vi "Main.vi"() -> ()   [LabVIEW 2018] (continued)
                n297 = case shown="真" w8265 {
                  tunnel: w8264 -> [_ w8271]
                  tunnel: w8263 -> [w8267 w8270]
                  tunnel: [w8267 w8269] -> _
                  frame False {
                  }
                  frame True {
                    n298 = flat-sequence {
                      tunnel: [w8274] -> w8272
                      tunnel: w8271 -> [w8273]
                      tunnel: w8270 -> [w8275]
                      tunnel: [w8273] -> w8268
                      tunnel: w8272 -> [w8305]
                      tunnel: [w8297] -> w8269
                      tunnel: w8268 -> [w8289]
                      frame #0 {
                        n299 = call "EXCEL 画曲线.vi"("错误输入（无错误）"=w8275, "路径"=w8273) -> ("error IO"=w8274:errorcluster, "XY图"=→"ST70_R曲线":cluster{"X":dbl, "Y":dbl}[])  [unwired: 6 in, 2 out]
                      }
                      frame #1 {
                        w8285 = path "D:/Data_Storage/temp" ("appended path")
                        n300 = local read "70编码"() -> (w8284:string)
                        n301 = call <vilib>:"Check if File or Folder Exists.vi"("path"=w8285) -> ("error out"=w8299:errorcluster, "file or folder exists?"=w8298:bool)  [unwired: 8 in, 1 out]
                        n302 = case shown="假" w8298 {
                          tunnel: w8285 -> [w8322 w8324]
                          tunnel: [w8321 w8324] -> w8291
                          tunnel: w8299 -> [w8320 w8323]
                          tunnel: [w8319 w8323] -> w8292
                          frame False {
                            n303 = Create Folder(path (use dialog)=w8322, error in=w8320) -> (created path=w8321:path, error out=w8319:errorcluster)  [unwired: 1 in, 1 out]
                          }
                          frame True {
                          }
                        }
                        n304 = Concatenate Strings(w8284, "ST70_R.BMP" ("字符串")) -> (w8302:string)
                        n305 = Build Path(base path=w8291, name or relative path=w8284) -> (appended path=w8293:path)
                        n306 = call <vilib>:"Check if File or Folder Exists.vi"("error in (no error)"=w8292, "path"=w8293) -> ("error out"=w8294:errorcluster, "file or folder exists?"=w8295:bool)  [unwired: 7 in, 1 out]
                        n307 = case shown="假" w8295 {
                          tunnel: w8293 -> [w8316 w8318]
                          tunnel: [w8315 w8318] -> w8280
                          tunnel: w8294 -> [w8314 w8317]
                          tunnel: [w8313 w8317] -> w8278
                          frame False {
                            n308 = Create Folder(path (use dialog)=w8316, error in=w8314) -> (created path=w8315:path, error out=w8313:errorcluster)  [unwired: 1 in, 1 out]
                          }
                          frame True {
                          }
                        }
                        n309 = Build Path(base path=w8280, name or relative path="ST70R" ("名称或相对路径")) -> (appended path=w8283:path)
                        n310 = call <vilib>:"Check if File or Folder Exists.vi"("error in (no error)"=w8278, "path"=w8283) -> ("error out"=w8282:errorcluster, "file or folder exists?"=w8281:bool)  [unwired: 7 in, 1 out]
                        n311 = case shown="假" w8281 {
                          tunnel: w8283 -> [w8310 w8312]
                          tunnel: [w8309 w8312] -> w8277
                          tunnel: w8282 -> [w8308 w8311]
                          tunnel: [w8307 w8311] -> _
                          frame False {
                            n312 = Create Folder(path (use dialog)=w8310, error in=w8308) -> (created path=w8309:path, error out=w8307:errorcluster)  [unwired: 1 in, 1 out]
                          }
                          frame True {
                          }
                        }
                        n313 = Build Path(base path=w8277, name or relative path=w8302) -> (appended path=w8288:path)
                        n314 = call "文件路径.vi"("文件路径"=w8288, "文件格式"=".BMP") -> ("新路径"=w8287:path)  [unwired: 9 in]
                        n315 = invoke on="ST70_R曲线" class="XYGraph (严格)" method="Export Image"(error in=w8305, "FileType"=enum32{"BMP", "EPS", "EMF", "PICT"}."BMP" ("文件类型"), "Target"=enum32{"File", "Clipboard"}."File" ("目标"), "Path"=w8287, "HideGrid"=FALSE ("隐藏网格"), "Overwrite"=TRUE ("隐藏网格")) -> (error out=w8290:errorcluster)  [unwired: 2 in, 7 out]
                        n316 = Move(source path=w8289, error in=w8290, 9:TRUE ("覆盖(F)"), 10:w8277) -> (error out=w8297:errorcluster)  [unwired: 1 in, 2 out]
                      }
                    }
                  }
                }
              }
              frame #1 {
                n317 = call "检查曲线文件.vi"("Folder Path"=path "D:/op70" ("路径")) -> ("Error Out"=w8327:errorcluster, "Exit?"=w8329:bool, "曲线文件路径"=w8328:path)  [unwired: 7 in, 1 out]
                n318 = case shown="真" w8329 {
                  tunnel: w8328 -> [_ w8334]
                  tunnel: w8327 -> [w8330 w8333]
                  tunnel: [w8330 w8332] -> w8325
                  frame False {
                  }
                  frame True {
                    n319 = flat-sequence {
                      tunnel: [w8337] -> w8335
                      tunnel: w8334 -> [w8336]
                      tunnel: w8333 -> [w8338]
                      tunnel: [w8336] -> w8331
                      tunnel: w8335 -> [w8369]
                      tunnel: [w8364] -> w8332
                      tunnel: w8331 -> [w8361]
                      frame #0 {
                        n320 = call "EXCEL 画曲线.vi"("错误输入（无错误）"=w8338, "路径"=w8336) -> ("error IO"=w8337:errorcluster, "XY图"=→"ST70_L曲线":cluster{"X":dbl, "Y":dbl}[])  [unwired: 6 in, 2 out]
                      }
                      frame #1 {
                        w8352 = path "D:/Data_Storage/temp" ("appended path")
                        n321 = local read "70编码"() -> (w8351:string)
                        n322 = call <vilib>:"Check if File or Folder Exists.vi"("path"=w8352) -> ("error out"=w8359:errorcluster, "file or folder exists?"=w8358:bool)  [unwired: 8 in, 1 out]
                        n323 = case shown="假" w8358 {
                          tunnel: w8352 -> [w8385 w8387]
                          tunnel: [w8384 w8387] -> w8353
                          tunnel: w8359 -> [w8383 w8386]
                          tunnel: [w8382 w8386] -> w8354
                          frame False {
                            n324 = Create Folder(path (use dialog)=w8385, error in=w8383) -> (created path=w8384:path, error out=w8382:errorcluster)  [unwired: 1 in, 1 out]
                          }
                          frame True {
                          }
                        }
                        n325 = Concatenate Strings(w8351, "ST70_L.BMP" ("字符串")) -> (w8340:string)
                        n326 = Build Path(base path=w8353, name or relative path=w8351) -> (appended path=w8355:path)
                        n327 = call <vilib>:"Check if File or Folder Exists.vi"("error in (no error)"=w8354, "path"=w8355) -> ("error out"=w8356:errorcluster, "file or folder exists?"=w8357:bool)  [unwired: 7 in, 1 out]
                        n328 = case shown="假" w8357 {
                          tunnel: w8355 -> [w8379 w8381]
                          tunnel: [w8378 w8381] -> w8347
                          tunnel: w8356 -> [w8377 w8380]
                          tunnel: [w8376 w8380] -> w8345
                          frame False {
                            n329 = Create Folder(path (use dialog)=w8379, error in=w8377) -> (created path=w8378:path, error out=w8376:errorcluster)  [unwired: 1 in, 1 out]
                          }
                          frame True {
                          }
                        }
                        n330 = Build Path(base path=w8347, name or relative path="ST70L" ("名称或相对路径")) -> (appended path=w8350:path)
                        n331 = call <vilib>:"Check if File or Folder Exists.vi"("error in (no error)"=w8345, "path"=w8350) -> ("error out"=w8349:errorcluster, "file or folder exists?"=w8348:bool)  [unwired: 7 in, 1 out]
                        n332 = case shown="假" w8348 {
                          tunnel: w8350 -> [w8373 w8375]
                          tunnel: [w8372 w8375] -> w8342
                          tunnel: w8349 -> [w8371 w8374]
                          tunnel: [w8370 w8374] -> _
                          frame False {
                            n333 = Create Folder(path (use dialog)=w8373, error in=w8371) -> (created path=w8372:path, error out=w8370:errorcluster)  [unwired: 1 in, 1 out]
                          }
                          frame True {
                          }
                        }
                        n334 = Build Path(base path=w8342, name or relative path=w8340) -> (appended path=w8344:path)
                        n335 = call "文件路径.vi"("文件路径"=w8344, "文件格式"=".BMP") -> ("新路径"=w8341:path)  [unwired: 9 in]
                        n336 = invoke on="ST70_L曲线" class="XYGraph (严格)" method="Export Image"(error in=w8369, "FileType"=enum32{"BMP", "EPS", "EMF", "PICT"}."BMP" ("文件类型"), "Target"=enum32{"File", "Clipboard"}."File" ("目标"), "Path"=w8341, "HideGrid"=FALSE ("隐藏网格"), "Overwrite"=TRUE ("隐藏网格")) -> (error out=w8362:errorcluster)  [unwired: 2 in, 7 out]
                        n337 = Move(source path=w8361, error in=w8362, 9:TRUE ("覆盖(F)"), 10:w8342) -> (error out=w8364:errorcluster)  [unwired: 1 in, 2 out]
                      }
                    }
                  }
                }
              }
            }
            n338 = case shown="错误" w8261 {
              selector: w8261 -> [_ w8396]
              frame No Error {
                w8390 = path "D:/op70" ("路径")
                n339 = List Folder(path=w8390) -> (filenames=w8391:string[])  [unwired: 3 in, 3 out]
                n340 = local write "数据保存请求回复70"("1" ("数据保存请求回复70")) -> ()
                n341 = local write "70数据回复输入"(TRUE) -> ()
                n342 = for {
                  tunnel: w8391 -> [w8394] mode=indexing
                  tunnel: w8390 -> [w8395]
                  n343 = Build Path(base path=w8395, name or relative path=w8394) -> (appended path=w8392:path)
                  n344 = Delete(path (use dialog)=w8392, entire hierarchy (F)=TRUE ("整个层次结构(F)")) -> ()  [unwired: 3 in, 3 out]
                }
              }
              frame Error {
                n345 = stacked-sequence {
                  tunnel: w8396 -> [w8402]
                  frame #0 {
                    n346 = Unbundle By Name(w8402) -> ("source"=w8401:string)
                    n347 = local write "数据保存请求回复70"("1" ("数据保存请求回复70")) -> ()
                    n348 = property on="错误信息" class="LstBox (严格)"() -> ("Item Names"=w8408:string[])  [unwired: 2 in, 2 out]
                    n349 = Format Date/Time String(time format string (%c)="%Y-%m-%d %H:%M:%S" ("时间格式字符串(%c)")) -> (date/time string=w8403:string)  [unwired: 2 in]
                    n350 = Concatenate Strings(w8403, "---" ("字符串"), w8401) -> (w8399:string)
                    n351 = Concatenate Strings(w8399, "  " ("字符串"), "ST70 画曲线错误") -> (w8406:string)
                    n352 = local write "70数据回复输入"(TRUE) -> ()
                    n353 = Insert Into Array(array=w8408, index=0 ("索引"), new element=w8406) -> (w8405:string[])
                    n354 = property on="错误信息" class="LstBox (严格)"("Item Names"=w8405) -> ()  [unwired: 2 in, 2 out]
                  }
                }
              }
            }
            "ST70画曲线" <- FALSE ("ST70画曲线")
          }
          event "ST90画曲线": Value Change {
            n355 = event-data() -> ()  [unwired: 1 in, 3 out]
            n356 = stacked-sequence {
              seq-local: [w8413 _ _ _ _ _] -> [_ _ _ _ _ w8717]
              seq-local: [_ w8481 _ _ _ _] -> [_ _ _ _ _ w8716]
              seq-local: [_ _ w8539 _ _ _] -> [_ _ _ _ _ w8715]
              seq-local: [_ _ _ w8597 _ _] -> [_ _ _ _ _ w8714]
              seq-local: [_ _ _ _ w8655 _] -> [_ _ _ _ _ w8713]
              frame #0 {
                w8415 = "ST70R" ("名称或相对路径")
                w8417 = path "D:/Data_Storage/temp" ("appended path")
                w8420 = path "D:/Data_Storage/temp" ("appended path")
                n357 = local read "901二维码"() -> (w8434:string)
                n358 = call "图片保存.vi"("一维码"=w8434) -> ("dup path"=w8435:path)  [unwired: 9 in, 1 out]
                n359 = Build Path(base path=w8435, name or relative path=w8434) -> (appended path=w8431:path)
                n360 = call <vilib>:"Check if File or Folder Exists.vi"("path"=w8431) -> ("error out"=w8433:errorcluster, "file or folder exists?"=w8432:bool)  [unwired: 8 in, 1 out]
                n361 = case shown="假" w8432 {
                  tunnel: w8431 -> [w8478 w8480]
                  tunnel: [w8477 w8480] -> w8421
                  tunnel: w8433 -> [w8476 w8479]
                  tunnel: [w8475 w8479] -> w8426
                  frame False {
                    n362 = Create Folder(path (use dialog)=w8478, error in=w8476) -> (created path=w8477:path, error out=w8475:errorcluster)  [unwired: 1 in, 1 out]
                  }
                  frame True {
                  }
                }
                n363 = local read "901编码"() -> (w8419:string)
                n364 = Build Path(base path=w8420, name or relative path=w8419) -> (appended path=w8430:path)
                n365 = Build Path(base path=w8430, name or relative path="ST70L" ("名称或相对路径")) -> (appended path=w8427:path)
                n366 = Move(source path=w8427, error in=w8426, 9:TRUE ("覆盖(F)"), 10:w8421) -> (error out=w8422:errorcluster)  [unwired: 1 in, 2 out]
                n367 = case shown="错误" w8422 {
                  tunnel: [errorcluster {"status"=FALSE, "code"=0, "source"=""} ("error out") w8460] -> w8412
                  tunnel: w8421 -> [w8455 w8457]
                  tunnel: w8420 -> [_ w8459]
                  tunnel: w8419 -> [_ w8458]
                  tunnel: [w8455 w8457] -> w8414
                  frame No Error {
                  }
                  frame Error {
                    n368 = Build Path(base path=w8459, name or relative path=w8458) -> (appended path=w8464:path)
                    n369 = Build Path(base path=w8464, name or relative path="ST70L" ("名称或相对路径")) -> (appended path=w8461:path)
                    n370 = Move(source path=w8461, 9:TRUE ("覆盖(F)"), 10:w8457) -> (error out=w8460:errorcluster)  [unwired: 2 in, 2 out]
                  }
                }
                n371 = local read "901编码"() -> (w8416:string)
                n372 = Build Path(base path=w8417, name or relative path=w8416) -> (appended path=w8425:path)
                n373 = Build Path(base path=w8425, name or relative path=w8415) -> (appended path=w8423:path)
                n374 = Move(source path=w8423, 9:TRUE ("覆盖(F)"), 10:w8414) -> (error out=w8418:errorcluster)  [unwired: 2 in, 2 out]
                n375 = case shown="错误" w8418 {
                  tunnel: w8417 -> [_ w8453]
                  tunnel: w8416 -> [_ w8452]
                  tunnel: w8415 -> [_ w8451]
                  tunnel: w8414 -> [_ w8448]
                  tunnel: [errorcluster {"status"=FALSE, "code"=0, "source"=""} ("error out") w8447] -> w8413
                  frame No Error {
                  }
                  frame Error {
                    n376 = Build Path(base path=w8453, name or relative path=w8452) -> (appended path=w8454:path)
                    n377 = Build Path(base path=w8454, name or relative path=w8451) -> (appended path=w8450:path)
                    n378 = Move(source path=w8450, 9:TRUE ("覆盖(F)"), 10:w8448) -> (error out=w8447:errorcluster)  [unwired: 2 in, 2 out]
                  }
                }
                n379 = case shown="错误" w8413 {
                  selector: w8413 -> [_ w8466]
                  frame No Error {
                  }
                  frame Error {
                    w8467 = "  " ("字符串")
                    n380 = Unbundle By Name(w8466) -> ("source"=w8465:string)
                    n381 = property on="错误信息" class="LstBox (严格)"() -> ("Item Names"=w8472:string[])  [unwired: 2 in, 2 out]
                    n382 = Format Date/Time String(time format string (%c)="%Y-%m-%d %H:%M:%S" ("时间格式字符串(%c)")) -> (date/time string=w8473:string)  [unwired: 2 in]
                    n383 = Concatenate Strings(w8473, w8467, "ST90 转移曲线失败ST70R", w8467, w8465) -> (w8470:string)
                    n384 = Insert Into Array(array=w8472, index=0 ("索引"), new element=w8470) -> (w8469:string[])
                    n385 = property on="错误信息" class="LstBox (严格)"("Item Names"=w8469) -> ()  [unwired: 2 in, 2 out]
                  }
                }
                n386 = case shown="错误" w8412 {
                  selector: w8412 -> [_ w8439]
                  frame No Error {
                  }
                  frame Error {
                    w8440 = "  " ("字符串")
                    n387 = Unbundle By Name(w8439) -> ("source"=w8438:string)
                    n388 = property on="错误信息" class="LstBox (严格)"() -> ("Item Names"=w8437:string[])  [unwired: 2 in, 2 out]
                    n389 = Format Date/Time String(time format string (%c)="%Y-%m-%d %H:%M:%S" ("时间格式字符串(%c)")) -> (date/time string=w8444:string)  [unwired: 2 in]
                    n390 = Concatenate Strings(w8444, w8440, "ST90 转移曲线失败ST70L", w8440, w8438) -> (w8442:string)
                    n391 = Insert Into Array(array=w8437, index=0 ("索引"), new element=w8442) -> (w8436:string[])
                    n392 = property on="错误信息" class="LstBox (严格)"("Item Names"=w8436) -> ()  [unwired: 2 in, 2 out]
                  }
                }
              }
              frame #1 {
                n393 = flat-sequence {
                  tunnel: [w8485] -> w8483
                  tunnel: [w8484] -> w8482
                  tunnel: w8483 -> [w8493]
                  tunnel: w8482 -> [w8502]
                  tunnel: [w8491] -> w8481
                  frame #0 {
                    n394 = local read "901二维码"() -> (w8484:string)
                    n395 = Concatenate Strings("D:\\BOSCH\\OP90\\CH_00_1\\PRG_00\\Ch_", w8484, "_001", "______.txt" ("字符串")) -> (w8488:string)
                    n396 = String To Path(string=w8488) -> (path=w8485:path)
                    n397 = call "140画曲线.vi"("文件（使用对话框）"=w8485) -> ("压机旋铆位移压力图"=→"压机旋铆位移压力图_1":cluster{dbl[], dbl[]})  [unwired: 10 in]
                  }
                  frame #1 {
                    n398 = call "图片保存.vi"("一维码"=w8502) -> ("dup path"=w8503:path)  [unwired: 9 in, 1 out]
                    n399 = Build Path(base path=w8503, name or relative path=w8502) -> (appended path=w8518:path)
                    n400 = call <vilib>:"Check if File or Folder Exists.vi"("path"=w8518) -> ("error out"=w8516:errorcluster, "file or folder exists?"=w8517:bool)  [unwired: 8 in, 1 out]
                    n401 = case shown="假" w8517 {
                      tunnel: w8518 -> [w8536 w8538]
                      tunnel: [w8535 w8538] -> w8512
                      tunnel: w8516 -> [w8534 w8537]
                      tunnel: [w8533 w8537] -> w8510
                      frame False {
                        n402 = Create Folder(path (use dialog)=w8536, error in=w8534) -> (created path=w8535:path, error out=w8533:errorcluster)  [unwired: 1 in, 1 out]
                      }
                      frame True {
                      }
                    }
                    n403 = Build Path(base path=w8512, name or relative path="ST901" ("名称或相对路径")) -> (appended path=w8513:path)
                    n404 = call <vilib>:"Check if File or Folder Exists.vi"("error in (no error)"=w8510, "path"=w8513) -> ("error out"=w8514:errorcluster, "file or folder exists?"=w8515:bool)  [unwired: 7 in, 1 out]
                    n405 = case shown="假" w8515 {
                      tunnel: w8513 -> [w8530 w8532]
                      tunnel: [w8529 w8532] -> w8507
                      tunnel: w8514 -> [w8528 w8531]
                      tunnel: [w8527 w8531] -> w8501
                      frame False {
                        n406 = Create Folder(path (use dialog)=w8530, error in=w8528) -> (created path=w8529:path, error out=w8527:errorcluster)  [unwired: 1 in, 1 out]
                      }
                      frame True {
                      }
                    }
                    n407 = Concatenate Strings("Ch_" ("字符串"), w8502, "_001______.txt" ("字符串")) -> (w8504:string)
                    n408 = Concatenate Strings(w8502, "_ST901_001.BMP" ("字符串")) -> (w8508:string)
                    n409 = Build Path(base path=w8507, name or relative path=w8508) -> (appended path=w8498:path)
                    n410 = Build Path(base path=w8507, name or relative path=w8504) -> (appended path=w8492:path)
                    n411 = invoke on="压机旋铆位移压力图_1" class="XYGraph (严格)" method="Export Image"(error in=w8501, "FileType"=enum32{"BMP", "EPS", "EMF", "PICT"}."BMP" ("文件类型"), "Target"=enum32{"File", "Clipboard"}."File" ("目标"), "Path"=w8498, "HideGrid"=FALSE ("隐藏网格"), "Overwrite"=TRUE ("始终覆盖")) -> (error out=w8494:errorcluster)  [unwired: 2 in, 7 out]
                    n412 = Move(source path=w8493, error in=w8494, 9:TRUE ("覆盖(F)"), 10:w8492) -> (error out=w8491:errorcluster)  [unwired: 1 in, 2 out]
                    n413 = case shown="错误" w8491 {
                      frame No Error {
                      }
                      frame Error {
                        n414 = property on="错误信息" class="LstBox (严格)"() -> ("Item Names"=w8523:string[])  [unwired: 2 in, 2 out]
                        n415 = Format Date/Time String(time format string (%c)="%Y-%m-%d %H:%M:%S" ("时间格式字符串(%c)")) -> (date/time string=w8525:string)  [unwired: 2 in]
                        n416 = Concatenate Strings(w8525, "  " ("字符串"), "ST901 画曲线错误") -> (w8521:string)
                        n417 = Insert Into Array(array=w8523, index=0 ("索引"), new element=w8521) -> (w8520:string[])
                        n418 = property on="错误信息" class="LstBox (严格)"("Item Names"=w8520) -> ()  [unwired: 2 in, 2 out]
                      }
                    }
                  }
                }
              }
              frame #2 {
                n419 = flat-sequence {
                  tunnel: [w8543] -> w8541
                  tunnel: [w8542] -> w8540
                  tunnel: w8541 -> [w8551]
                  tunnel: w8540 -> [w8560]
                  tunnel: [w8549] -> w8539
                  frame #0 {
                    n420 = local read "901二维码"() -> (w8542:string)
                    n421 = Concatenate Strings("D:\\BOSCH\\OP90\\CH_00_1\\PRG_00\\Ch_", w8542, "_002", "______.txt" ("字符串")) -> (w8546:string)
                    n422 = String To Path(string=w8546) -> (path=w8543:path)
                    n423 = call "140画曲线.vi"("文件（使用对话框）"=w8543) -> ("压机旋铆位移压力图"=→"压机旋铆位移压力图_2":cluster{dbl[], dbl[]})  [unwired: 10 in]
                  }
                  frame #1 {
                    n424 = call "图片保存.vi"("一维码"=w8560) -> ("dup path"=w8561:path)  [unwired: 9 in, 1 out]
                    n425 = Build Path(base path=w8561, name or relative path=w8560) -> (appended path=w8576:path)
                    n426 = call <vilib>:"Check if File or Folder Exists.vi"("path"=w8576) -> ("error out"=w8574:errorcluster, "file or folder exists?"=w8575:bool)  [unwired: 8 in, 1 out]
                    n427 = case shown="假" w8575 {
                      tunnel: w8576 -> [w8594 w8596]
                      tunnel: [w8593 w8596] -> w8570
                      tunnel: w8574 -> [w8592 w8595]
                      tunnel: [w8591 w8595] -> w8568
                      frame False {
                        n428 = Create Folder(path (use dialog)=w8594, error in=w8592) -> (created path=w8593:path, error out=w8591:errorcluster)  [unwired: 1 in, 1 out]
                      }
                      frame True {
                      }
                    }
                    n429 = Build Path(base path=w8570, name or relative path="ST901" ("名称或相对路径")) -> (appended path=w8571:path)
                    n430 = call <vilib>:"Check if File or Folder Exists.vi"("error in (no error)"=w8568, "path"=w8571) -> ("error out"=w8572:errorcluster, "file or folder exists?"=w8573:bool)  [unwired: 7 in, 1 out]
                    n431 = case shown="假" w8573 {
                      tunnel: w8571 -> [w8588 w8590]
                      tunnel: [w8587 w8590] -> w8565
                      tunnel: w8572 -> [w8586 w8589]
                      tunnel: [w8585 w8589] -> w8559
                      frame False {
                        n432 = Create Folder(path (use dialog)=w8588, error in=w8586) -> (created path=w8587:path, error out=w8585:errorcluster)  [unwired: 1 in, 1 out]
                      }
                      frame True {
                      }
                    }
                    n433 = Concatenate Strings("Ch_" ("字符串"), w8560, "_002______.txt" ("字符串")) -> (w8562:string)
                    n434 = Concatenate Strings(w8560, "_ST901_002.BMP" ("字符串")) -> (w8566:string)
                    n435 = Build Path(base path=w8565, name or relative path=w8566) -> (appended path=w8556:path)
                    n436 = Build Path(base path=w8565, name or relative path=w8562) -> (appended path=w8550:path)
                    n437 = invoke on="压机旋铆位移压力图_2" class="XYGraph (严格)" method="Export Image"(error in=w8559, "FileType"=enum32{"BMP", "EPS", "EMF", "PICT"}."BMP" ("文件类型"), "Target"=enum32{"File", "Clipboard"}."File" ("目标"), "Path"=w8556, "HideGrid"=FALSE ("隐藏网格"), "Overwrite"=TRUE ("始终覆盖")) -> (error out=w8552:errorcluster)  [unwired: 2 in, 7 out]
                    n438 = Move(source path=w8551, error in=w8552, 9:TRUE ("覆盖(F)"), 10:w8550) -> (error out=w8549:errorcluster)  [unwired: 1 in, 2 out]
                    n439 = case shown="错误" w8549 {
                      frame No Error {
                      }
                      frame Error {
                        n440 = property on="错误信息" class="LstBox (严格)"() -> ("Item Names"=w8581:string[])  [unwired: 2 in, 2 out]
                        n441 = Format Date/Time String(time format string (%c)="%Y-%m-%d %H:%M:%S" ("时间格式字符串(%c)")) -> (date/time string=w8583:string)  [unwired: 2 in]
                        n442 = Concatenate Strings(w8583, "  " ("字符串"), "ST901 画曲线错误") -> (w8579:string)
                        n443 = Insert Into Array(array=w8581, index=0 ("索引"), new element=w8579) -> (w8578:string[])
                        n444 = property on="错误信息" class="LstBox (严格)"("Item Names"=w8578) -> ()  [unwired: 2 in, 2 out]
                      }
                    }
                  }
                }
              }
              frame #3 {
                n445 = flat-sequence {
                  tunnel: [w8601] -> w8599
                  tunnel: [w8600] -> w8598
                  tunnel: w8599 -> [w8609]
                  tunnel: w8598 -> [w8618]
                  tunnel: [w8607] -> w8597
                  frame #0 {
                    n446 = local read "901二维码"() -> (w8600:string)
                    n447 = Concatenate Strings("D:\\BOSCH\\OP90\\CH_00_1\\PRG_00\\Ch_", w8600, "_003", "______.txt" ("字符串")) -> (w8604:string)
                    n448 = String To Path(string=w8604) -> (path=w8601:path)
                    n449 = call "140画曲线.vi"("文件（使用对话框）"=w8601) -> ("压机旋铆位移压力图"=→"压机旋铆位移压力图_3":cluster{dbl[], dbl[]})  [unwired: 10 in]
                  }
                  frame #1 {
                    n450 = call "图片保存.vi"("一维码"=w8618) -> ("dup path"=w8619:path)  [unwired: 9 in, 1 out]
                    n451 = Build Path(base path=w8619, name or relative path=w8618) -> (appended path=w8634:path)
                    n452 = call <vilib>:"Check if File or Folder Exists.vi"("path"=w8634) -> ("error out"=w8632:errorcluster, "file or folder exists?"=w8633:bool)  [unwired: 8 in, 1 out]
                    n453 = case shown="假" w8633 {
                      tunnel: w8634 -> [w8652 w8654]
                      tunnel: [w8651 w8654] -> w8628
                      tunnel: w8632 -> [w8650 w8653]
                      tunnel: [w8649 w8653] -> w8626
                      frame False {
                        n454 = Create Folder(path (use dialog)=w8652, error in=w8650) -> (created path=w8651:path, error out=w8649:errorcluster)  [unwired: 1 in, 1 out]
                      }
                      frame True {
                      }
                    }
                    n455 = Build Path(base path=w8628, name or relative path="ST901" ("名称或相对路径")) -> (appended path=w8629:path)
                    n456 = call <vilib>:"Check if File or Folder Exists.vi"("error in (no error)"=w8626, "path"=w8629) -> ("error out"=w8630:errorcluster, "file or folder exists?"=w8631:bool)  [unwired: 7 in, 1 out]
                    n457 = case shown="假" w8631 {
                      tunnel: w8629 -> [w8646 w8648]
                      tunnel: [w8645 w8648] -> w8623
                      tunnel: w8630 -> [w8644 w8647]
                      tunnel: [w8643 w8647] -> w8617
                      frame False {
                        n458 = Create Folder(path (use dialog)=w8646, error in=w8644) -> (created path=w8645:path, error out=w8643:errorcluster)  [unwired: 1 in, 1 out]
                      }
                      frame True {
                      }
                    }
                    n459 = Concatenate Strings("Ch_" ("字符串"), w8618, "_003______.txt" ("字符串")) -> (w8620:string)
                    n460 = Concatenate Strings(w8618, "_ST901_003.BMP" ("字符串")) -> (w8624:string)
                    n461 = Build Path(base path=w8623, name or relative path=w8624) -> (appended path=w8614:path)
                    n462 = Build Path(base path=w8623, name or relative path=w8620) -> (appended path=w8608:path)
                    n463 = invoke on="压机旋铆位移压力图_3" class="XYGraph (严格)" method="Export Image"(error in=w8617, "FileType"=enum32{"BMP", "EPS", "EMF", "PICT"}."BMP" ("文件类型"), "Target"=enum32{"File", "Clipboard"}."File" ("目标"), "Path"=w8614, "HideGrid"=FALSE ("隐藏网格"), "Overwrite"=TRUE ("始终覆盖")) -> (error out=w8610:errorcluster)  [unwired: 2 in, 7 out]
                    n464 = Move(source path=w8609, error in=w8610, 9:TRUE ("覆盖(F)"), 10:w8608) -> (error out=w8607:errorcluster)  [unwired: 1 in, 2 out]
                    n465 = case shown="错误" w8607 {
                      frame No Error {
                      }
                      frame Error {
                        n466 = property on="错误信息" class="LstBox (严格)"() -> ("Item Names"=w8639:string[])  [unwired: 2 in, 2 out]
                        n467 = Format Date/Time String(time format string (%c)="%Y-%m-%d %H:%M:%S" ("时间格式字符串(%c)")) -> (date/time string=w8641:string)  [unwired: 2 in]
                        n468 = Concatenate Strings(w8641, "  " ("字符串"), "ST901 画曲线错误") -> (w8637:string)
                        n469 = Insert Into Array(array=w8639, index=0 ("索引"), new element=w8637) -> (w8636:string[])
                        n470 = property on="错误信息" class="LstBox (严格)"("Item Names"=w8636) -> ()  [unwired: 2 in, 2 out]
                      }
                    }
                  }
                }
              }
              frame #4 {
                n471 = flat-sequence {
                  tunnel: [w8659] -> w8657
                  tunnel: [w8658] -> w8656
                  tunnel: w8657 -> [w8667]
                  tunnel: w8656 -> [w8676]
                  tunnel: [w8665] -> w8655
                  frame #0 {
                    n472 = local read "901二维码"() -> (w8658:string)
                    n473 = Concatenate Strings("D:\\BOSCH\\OP90\\CH_00_1\\PRG_00\\Ch_", w8658, "_004", "______.txt" ("字符串")) -> (w8662:string)
                    n474 = String To Path(string=w8662) -> (path=w8659:path)
                    n475 = call "140画曲线.vi"("文件（使用对话框）"=w8659) -> ("压机旋铆位移压力图"=→"压机旋铆位移压力图_4":cluster{dbl[], dbl[]})  [unwired: 10 in]
                  }
                  frame #1 {
                    n476 = call "图片保存.vi"("一维码"=w8676) -> ("dup path"=w8677:path)  [unwired: 9 in, 1 out]
                    n477 = Build Path(base path=w8677, name or relative path=w8676) -> (appended path=w8692:path)
                    n478 = call <vilib>:"Check if File or Folder Exists.vi"("path"=w8692) -> ("error out"=w8690:errorcluster, "file or folder exists?"=w8691:bool)  [unwired: 8 in, 1 out]
                    n479 = case shown="假" w8691 {
                      tunnel: w8692 -> [w8710 w8712]
                      tunnel: [w8709 w8712] -> w8686
                      tunnel: w8690 -> [w8708 w8711]
                      tunnel: [w8707 w8711] -> w8684
                      frame False {
                        n480 = Create Folder(path (use dialog)=w8710, error in=w8708) -> (created path=w8709:path, error out=w8707:errorcluster)  [unwired: 1 in, 1 out]
                      }
                      frame True {
                      }
                    }
                    n481 = Build Path(base path=w8686, name or relative path="ST901" ("名称或相对路径")) -> (appended path=w8687:path)
                    n482 = call <vilib>:"Check if File or Folder Exists.vi"("error in (no error)"=w8684, "path"=w8687) -> ("error out"=w8688:errorcluster, "file or folder exists?"=w8689:bool)  [unwired: 7 in, 1 out]
                    n483 = case shown="假" w8689 {
                      tunnel: w8687 -> [w8704 w8706]
                      tunnel: [w8703 w8706] -> w8681
                      tunnel: w8688 -> [w8702 w8705]
                      tunnel: [w8701 w8705] -> w8675
                      frame False {
                        n484 = Create Folder(path (use dialog)=w8704, error in=w8702) -> (created path=w8703:path, error out=w8701:errorcluster)  [unwired: 1 in, 1 out]
                      }
                      frame True {
                      }
                    }
                    n485 = Concatenate Strings("Ch_" ("字符串"), w8676, "_004______.txt" ("字符串")) -> (w8678:string)
                    n486 = Concatenate Strings(w8676, "_ST901_004.BMP" ("字符串")) -> (w8682:string)
                    n487 = Build Path(base path=w8681, name or relative path=w8682) -> (appended path=w8672:path)
                    n488 = Build Path(base path=w8681, name or relative path=w8678) -> (appended path=w8666:path)
                    n489 = invoke on="压机旋铆位移压力图_4" class="XYGraph (严格)" method="Export Image"(error in=w8675, "FileType"=enum32{"BMP", "EPS", "EMF", "PICT"}."BMP" ("文件类型"), "Target"=enum32{"File", "Clipboard"}."File" ("目标"), "Path"=w8672, "HideGrid"=FALSE ("隐藏网格"), "Overwrite"=TRUE ("始终覆盖")) -> (error out=w8668:errorcluster)  [unwired: 2 in, 7 out]
                    n490 = Move(source path=w8667, error in=w8668, 9:TRUE ("覆盖(F)"), 10:w8666) -> (error out=w8665:errorcluster)  [unwired: 1 in, 2 out]
                    n491 = case shown="错误" w8665 {
                      frame No Error {
                      }
                      frame Error {
                        n492 = property on="错误信息" class="LstBox (严格)"() -> ("Item Names"=w8697:string[])  [unwired: 2 in, 2 out]
                        n493 = Format Date/Time String(time format string (%c)="%Y-%m-%d %H:%M:%S" ("时间格式字符串(%c)")) -> (date/time string=w8699:string)  [unwired: 2 in]
                        n494 = Concatenate Strings(w8699, "  " ("字符串"), "ST901 画曲线错误") -> (w8695:string)
                        n495 = Insert Into Array(array=w8697, index=0 ("索引"), new element=w8695) -> (w8694:string[])
                        n496 = property on="错误信息" class="LstBox (严格)"("Item Names"=w8694) -> ()  [unwired: 2 in, 2 out]
                      }
                    }
                  }
                }
              }
              frame #5 {
                n497 = flat-sequence {
                  tunnel: [w8721] -> w8719
                  tunnel: [w8720] -> w8718
                  tunnel: w8719 -> [w8735]
                  tunnel: w8718 -> [w8744]
                  tunnel: w8717 -> [w8733]
                  tunnel: w8716 -> [w8732]
                  tunnel: w8715 -> [w8731]
                  tunnel: w8714 -> [w8730]
                  tunnel: w8713 -> [w8729]
                  frame #0 {
                    n498 = local read "901二维码"() -> (w8720:string)
                    n499 = Concatenate Strings("D:\\BOSCH\\OP90\\CH_00_1\\PRG_00\\Ch_", w8720, "_005", "______.txt" ("字符串")) -> (w8724:string)
                    n500 = String To Path(string=w8724) -> (path=w8721:path)
                    n501 = call "140画曲线.vi"("文件（使用对话框）"=w8721) -> ("压机旋铆位移压力图"=→"压机旋铆位移压力图_5":cluster{dbl[], dbl[]})  [unwired: 10 in]
                  }
                  frame #1 {
                    n502 = call "图片保存.vi"("一维码"=w8744) -> ("dup path"=w8745:path)  [unwired: 9 in, 1 out]
                    n503 = Build Path(base path=w8745, name or relative path=w8744) -> (appended path=w8760:path)
                    n504 = call <vilib>:"Check if File or Folder Exists.vi"("path"=w8760) -> ("error out"=w8758:errorcluster, "file or folder exists?"=w8759:bool)  [unwired: 8 in, 1 out]
                    n505 = case shown="假" w8759 {
                      tunnel: w8760 -> [w8782 w8784]
                      tunnel: [w8781 w8784] -> w8754
                      tunnel: w8758 -> [w8780 w8783]
                      tunnel: [w8779 w8783] -> w8752
                      frame False {
                        n506 = Create Folder(path (use dialog)=w8782, error in=w8780) -> (created path=w8781:path, error out=w8779:errorcluster)  [unwired: 1 in, 1 out]
                      }
                      frame True {
                      }
                    }
                    n507 = Build Path(base path=w8754, name or relative path="ST901" ("名称或相对路径")) -> (appended path=w8755:path)
                    n508 = call <vilib>:"Check if File or Folder Exists.vi"("error in (no error)"=w8752, "path"=w8755) -> ("error out"=w8756:errorcluster, "file or folder exists?"=w8757:bool)  [unwired: 7 in, 1 out]
                    n509 = case shown="假" w8757 {
                      tunnel: w8755 -> [w8776 w8778]
                      tunnel: [w8775 w8778] -> w8749
                      tunnel: w8756 -> [w8774 w8777]
                      tunnel: [w8773 w8777] -> w8743
                      frame False {
                        n510 = Create Folder(path (use dialog)=w8776, error in=w8774) -> (created path=w8775:path, error out=w8773:errorcluster)  [unwired: 1 in, 1 out]
                      }
                      frame True {
                      }
                    }
                    n511 = Concatenate Strings("Ch_" ("字符串"), w8744, "_005______.txt" ("字符串")) -> (w8746:string)
                    n512 = Concatenate Strings(w8744, "_ST901_005.BMP" ("字符串")) -> (w8750:string)
                    n513 = Build Path(base path=w8749, name or relative path=w8750) -> (appended path=w8740:path)
                    n514 = Build Path(base path=w8749, name or relative path=w8746) -> (appended path=w8734:path)
                    n515 = invoke on="压机旋铆位移压力图_5" class="XYGraph (严格)" method="Export Image"(error in=w8743, "FileType"=enum32{"BMP", "EPS", "EMF", "PICT"}."BMP" ("文件类型"), "Target"=enum32{"File", "Clipboard"}."File" ("目标"), "Path"=w8740, "HideGrid"=FALSE ("隐藏网格"), "Overwrite"=TRUE ("始终覆盖")) -> (error out=w8736:errorcluster)  [unwired: 2 in, 7 out]
                    n516 = Move(source path=w8735, error in=w8736, 9:TRUE ("覆盖(F)"), 10:w8734) -> (error out=w8728:errorcluster)  [unwired: 1 in, 2 out]
                    n517 = case shown="错误" w8728 {
                      frame No Error {
                      }
                      frame Error {
                        n518 = property on="错误信息" class="LstBox (严格)"() -> ("Item Names"=w8769:string[])  [unwired: 2 in, 2 out]
                        n519 = Format Date/Time String(time format string (%c)="%Y-%m-%d %H:%M:%S" ("时间格式字符串(%c)")) -> (date/time string=w8771:string)  [unwired: 2 in]
                        n520 = Concatenate Strings(w8771, "  " ("字符串"), "ST901 画曲线错误") -> (w8767:string)
                        n521 = Insert Into Array(array=w8769, index=0 ("索引"), new element=w8767) -> (w8766:string[])
                        n522 = property on="错误信息" class="LstBox (严格)"("Item Names"=w8766) -> ()  [unwired: 2 in, 2 out]
                      }
                    }
                    n523 = Merge Errors(w8729, w8730, w8731, w8732, w8733, w8728) -> (w8727:errorcluster)
                    n524 = case shown="错误" w8727 {
                      frame No Error {
                        n525 = local write "数据保存请求回复901"("1" ("数据保存请求回复901")) -> ()
                        n526 = local write "901数据回复输入"(TRUE ("901数据回复输入")) -> ()
                      }
                      frame Error {
                        n527 = local write "数据保存请求回复901"("2" ("数据保存请求回复901")) -> ()
                        n528 = local write "901数据回复输入"(TRUE ("901数据回复输入")) -> ()
                      }
                    }
                  }
                }
              }
            }
            "ST90画曲线" <- FALSE ("ST90画曲线")
          }
        }
        n529 = Wait (ms)(milliseconds to wait=u32 10 ("等待时间（毫秒）")) -> ()  [unwired: 1 out]
      }
      n530 = while {
        shift-right: [w52] -> _
        shift-left: errorcluster {"status"=FALSE, "code"=0, "source"=""} ("错误常量") -> [w55]
        shift-right: [w51] -> _
        shift-left: enum16{"初始化", "读", "写", "错误", "退出"}."初始化" -> [w56]
        shift-right: [w53] -> _
        shift-left: _ -> [w50]
        stop <- w49 stop-if-true
        n531 = local read "退出"() -> (w57:bool)
        n532 = case shown="假" w57 {
          tunnel: w56 -> [w58 _]
          tunnel: [w59 enum16{"初始化", "读", "写", "错误", "退出"}."退出"] -> w48
          tunnel: w55 -> [w60 _]
          frame False {
            n533 = case shown="错误" w60 {
              tunnel: [w61 enum16{"初始化", "读", "写", "错误", "退出"}."错误"] -> w59
              tunnel: w58 -> [w61 _]
              frame No Error {
              }
              frame Error {
              }
            }
          }
          frame True {
          }
        }
        n534 = Wait (ms)(milliseconds to wait=u32 100 ("等待时间（毫秒）")) -> ()  [unwired: 1 out]
        n535 = Wait (ms)(milliseconds to wait=u32 80 ("等待时间（毫秒）")) -> ()  [unwired: 1 out]
        n536 = case shown="\"初始化\", 默认" w48 {
          tunnel: [w66 w87 w134 refnum<k5> refnum ("TCP") refnum<k5> refnum ("TCP")] -> w53
          tunnel: [w64 w86 w133 errorcluster {"status"=FALSE, "code"=0, "source"=""} ("error out") errorcluster {"status"=FALSE, "code"=0, "source"=""} ("error out")] -> w52
          tunnel: [enum16{"初始化", "读", "写", "错误", "退出"}."读" enum16{"初始化", "读", "写", "错误", "退出"}."写" enum16{"初始化", "读", "写", "错误", "退出"}."读" enum16{"初始化", "读", "写", "错误", "退出"}."初始化" enum16{"初始化", "读", "写", "错误", "退出"}."退出"] -> w51
          tunnel: w50 -> [_ w95 w150 w199 w206]
          tunnel: [FALSE FALSE FALSE FALSE TRUE] -> w49
          frame "初始化", Default {
            w76 = u16 0 items=["byte", "word", "Dword"] ("数据类型")
            w74 = u8 132 items=["I/O (P)"=128, "Input (I)"=129, "Output (Q)"=130, "Bit Memory (M)"=131, "Data (DB)"=132, "Instance Data (DI)"=133, "Local Data (L)"=134, "Predecessor Local Data (VL)"=135] ("寄存器类型")
            w81 = u8 0 items=["S7-1200.200.200SMART"=0, "S7-300"=2, "S7-400"=3] ("PLC 系列")
            n537 = call "S7_Open.vi"("IP 地址"="192.168.1.108", "PLC 系列"=w81, "超时（MS）"=100) -> ("TCP"=w67:refnum<k5>, "error out"=w65:errorcluster)  [unwired: 10 in, 1 out]
            n538 = case shown="错误" w65 {
              tunnel: [FALSE TRUE] -> w77
              frame No Error {
              }
              frame Error {
              }
            }
            n539 = local write "ST100通讯状态"(w77) -> ()
            n540 = call "S7_Read.vi"("TCP"=w67, "DB #"=u16 20, "读取长度"=u16 13, "寄存器类型"=w74, "起始地址"=u32 10, "数据类型"=w76, "error in"=w65) -> ("TCP"=w66:refnum<k5>, "数据"=w71:u32[], "error out"=w69:errorcluster)  [unwired: 5 in, 1 out]
            n541 = To Unsigned Word Integer(number=w71) -> (unsigned 16bit integer=w70:u16[])
            n542 = call "还原为字符串.vi"("error in (no error)"=w69, "输入数组"=w70) -> ("error out"=w64:errorcluster, "字符串"=w68:string)  [unwired: 8 in]
            n543 = local write "100二维码"(w68) -> ()
          }
          frame "读" {
            w96 = u16 0 items=["byte", "word", "Dword"] ("数据类型")
            w98 = u8 132 items=["I/O (P)"=128, "Input (I)"=129, "Output (Q)"=130, "Bit Memory (M)"=131, "Data (DB)"=132, "Instance Data (DI)"=133, "Local Data (L)"=134, "Predecessor Local Data (VL)"=135] ("寄存器类型")
            n544 = call "S7_Read.vi"("TCP"=w95, "DB #"=u16 20, "读取长度"=u16 1, "寄存器类型"=w98, "起始地址"=u32 0, "数据类型"=w96) -> ("TCP"=w93:refnum<k5>, "数据"=w103:u32[], "读取成功"=w106:bool, "error out"=w92:errorcluster)  [unwired: 6 in]
            n545 = Not(x=w106) -> (.not. x?=→"ST100通讯状态":bool)
            n546 = Index Array(array=w103, index=0 ("索引")) -> (element=w104:u32)
            n547 = Number To Boolean Array(number=w104) -> (Boolean array=w105:bool[])
            n548 = Index Array(array=w105, index=0 ("索引")) -> (element=w88:bool)
            "ST100扫码请求" <- w88
            n549 = disable-structure shown="启用" {
              disable-tunnel: [w109 w111] -> w90
              disable-tunnel: w88 -> [w108 w111]
              frame Disabled {
                n550 = call <vilib>:"Boolean Crossing PtByPt.vi"("direction"=enum16{"either", "false-true", "true-false"}."true-false", "input"=w108) -> ("crossing"=w109:bool)  [unwired: 1 in]
              }
              frame Enabled {
              }
            }
            n551 = call <vilib>:"Boolean Crossing PtByPt.vi"("direction"=enum16{"either", "false-true", "true-false"}."false-true", "input"=w88) -> ("crossing"=w91:bool)  [unwired: 1 in]
            n552 = case shown="真" w91 {
              tunnel: w93 -> [w114 w119]
              tunnel: w92 -> [w113 w120]
              tunnel: [w114 w118] -> w87
              tunnel: [w113 w116] -> w86
              frame False {
              }
              frame True {
                w128 = u16 0 items=["byte", "word", "Dword"] ("数据类型")
                w126 = u8 132 items=["I/O (P)"=128, "Input (I)"=129, "Output (Q)"=130, "Bit Memory (M)"=131, "Data (DB)"=132, "Instance Data (DI)"=133, "Local Data (L)"=134, "Predecessor Local Data (VL)"=135] ("寄存器类型")
                n553 = call "S7_Read.vi"("TCP"=w119, "DB #"=u16 20, "读取长度"=u16 13, "寄存器类型"=w126, "起始地址"=u32 10, "数据类型"=w128, "error in"=w120) -> ("TCP"=w118:refnum<k5>, "数据"=w123:u32[], "error out"=w121:errorcluster)  [unwired: 5 in, 1 out]
                n554 = To Unsigned Word Integer(number=w123) -> (unsigned 16bit integer=w122:u16[])
                n555 = call "还原为字符串.vi"("error in (no error)"=w121, "输入数组"=w122) -> ("error out"=w117:errorcluster, "字符串"=w115:string)  [unwired: 8 in]
                n556 = stacked-sequence {
                  tunnel: w117 -> [_ w132]
                  tunnel: [_ w131] -> w116
                  tunnel: w115 -> [w129 _]
                  frame #0 {
                    "100二维码" <- w129
                  }
                  frame #1 {
                    n557 = property on="ST100扫码请求（事件）" class="Bool (严格)"(error in=w132, "Val(Sgnl)"=TRUE ("值(信号)")) -> (error out=w131:errorcluster)  [unwired: 1 in, 1 out]
                  }
                }
              }
            }
            n558 = case shown="假" w90 {
              frame False {
                n559 = local write "100扫码回复输入"(FALSE ("301扫码回复输入")) -> ()
              }
              frame True {
              }
            }
          }
          frame "写" {
            w147 = u8 132 items=["I/O (P)"=128, "Input (I)"=129, "Output (Q)"=130, "Bit Memory (M)"=131, "Data (DB)"=132, "Instance Data (DI)"=133, "Local Data (L)"=134, "Predecessor Local Data (VL)"=135] ("寄存器类型")
            w146 = u16 1 items=["byte", "word", "Dword"] ("数据类型")
            w154 = u8 132 items=["I/O (P)"=128, "Input (I)"=129, "Output (Q)"=130, "Bit Memory (M)"=131, "Data (DB)"=132, "Instance Data (DI)"=133, "Local Data (L)"=134, "Predecessor Local Data (VL)"=135] ("寄存器类型")
            w151 = u16 1 items=["byte", "word", "Dword"] ("数据类型")
            n560 = local read "100看门狗"() -> (w140:i32)
            n561 = case shown="0" w140 {
              tunnel: [0 ("y") 1 ("y")] -> w137
              frame 1, Default {
              }
              frame 0 {
              }
            }
            "100看门狗" <- w137
            "100看门狗 2" <- w137
            n562 = call "S7_Write.vi"("TCP"=w150, "寄存器类型"=w154, "DB #"=u16 20, "写入地址"=u32 8, "数据类型"=w151, "写入数据"=w137) -> ("TCP"=w145:refnum<k5>, "error out"=w144:errorcluster)  [unwired: 7 in, 1 out]
            n563 = case shown="真" "100扫码回复输入" {
              tunnel: w145 -> [w169 w177]
              tunnel: w144 -> [w168 w176]
              tunnel: [w169 w175] -> w143
              tunnel: [w168 w174] -> w142
              tunnel: [999 w173] -> w141
              frame False {
              }
              frame True {
                w185 = u8 132 items=["I/O (P)"=128, "Input (I)"=129, "Output (Q)"=130, "Bit Memory (M)"=131, "Data (DB)"=132, "Instance Data (DI)"=133, "Local Data (L)"=134, "Predecessor Local Data (VL)"=135] ("寄存器类型")
                w184 = u16 1 items=["byte", "word", "Dword"] ("数据类型")
                w179 = u8 132 items=["I/O (P)"=128, "Input (I)"=129, "Output (Q)"=130, "Bit Memory (M)"=131, "Data (DB)"=132, "Instance Data (DI)"=133, "Local Data (L)"=134, "Predecessor Local Data (VL)"=135] ("寄存器类型")
                w180 = u16 1 items=["byte", "word", "Dword"] ("数据类型")
                n564 = local read "上一站号 (100)"() -> (w172:string)
                n565 = local read "上一站结果 (100)"() -> (w171:string)
                n566 = Decimal String To Number(string=w172, default (0L)=u32 0 ("默认(0 I32)")) -> (number=w189:u32)  [unwired: 1 in, 1 out]
                n567 = call "S7_Write.vi"("TCP"=w177, "寄存器类型"=w179, "DB #"=u16 20, "写入地址"=u32 4, "数据类型"=w180, "写入数据"=w189, "error in"=w176) -> ("TCP"=w188:refnum<k5>, "error out"=w187:errorcluster)  [unwired: 6 in, 1 out]
                n568 = Equal?(x=w171, y="OK") -> (x = y?=w191:bool)
                n569 = case shown="假" w191 {
                  tunnel: [u32 2 ("写入数据") u32 1 ("写入数据")] -> w192
                  frame False {
                  }
                  frame True {
                  }
                }
                n570 = local read "扫码请求回复100"() -> (w170:string)
                n571 = call "S7_Write.vi"("TCP"=w188, "寄存器类型"=w185, "DB #"=u16 20, "写入地址"=u32 6, "数据类型"=w184, "写入数据"=w192, "error in"=w187) -> ("TCP"=w175:refnum<k5>, "error out"=w174:errorcluster)  [unwired: 6 in, 1 out]
                n572 = Decimal String To Number(string=w170) -> (number=w173:i32)  [unwired: 2 in, 1 out]
              }
            }
            n573 = call "S7_Write.vi"("TCP"=w143, "寄存器类型"=w147, "DB #"=u16 20, "写入地址"=u32 2, "数据类型"=w146, "写入数据"=w141, "error in"=w142) -> ("TCP"=w136:refnum<k5>, "error out"=w135:errorcluster)  [unwired: 6 in, 1 out]
            n574 = disable-structure shown="启用" {
              disable-tunnel: w136 -> [w156 w160]
              disable-tunnel: [w156 w163] -> w134
              disable-tunnel: w135 -> [w157 w161]
              disable-tunnel: [w157 w162] -> w133
              frame Disabled {
              }
              frame Enabled {
                w165 = u8 132 items=["I/O (P)"=128, "Input (I)"=129, "Output (Q)"=130, "Bit Memory (M)"=131, "Data (DB)"=132, "Instance Data (DI)"=133, "Local Data (L)"=134, "Predecessor Local Data (VL)"=135] ("寄存器类型")
                w159 = u16 1 items=["byte", "word", "Dword"] ("数据类型")
                n575 = local read "产品型号"() -> (w158:u32)
                n576 = call "S7_Write.vi"("TCP"=w160, "寄存器类型"=w165, "DB #"=u16 20, "写入地址"=u32 24, "数据类型"=w159, "写入数据"=w158, "error in"=w161) -> ("TCP"=w163:refnum<k5>, "error out"=w162:errorcluster)  [unwired: 6 in, 1 out]
              }
            }
          }
          frame "错误" {
            n577 = call "S7_Close.vi"("TCP Connection Ref"=w199) -> ("error out"=w200:errorcluster)  [unwired: 10 in]
            n578 = call <vilib>:"Clear Errors.vi"("error in (no error)"=w200) -> ()  [unwired: 5 in, 2 out]
          }
          frame "退出" {
            n579 = call "S7_Close.vi"("TCP Connection Ref"=w206) -> ("error out"=w207:errorcluster)  [unwired: 10 in]
            n580 = call <vilib>:"Clear Errors.vi"("error in (no error)"=w207) -> ()  [unwired: 5 in, 2 out]
          }
        }
      }
      n581 = while {
        tunnel: w35 -> [w4421]
        tunnel: w36 -> [w4420]
        stop <- w4419 stop-if-true
        # "原50"
        n582 = event shown="[20] \"ST502扫码请求（事件）\": 值改变" {
          selector: _ -> [_ _ _ _ _ _ _ _ _ _ _ _ _ _ _ _ _ _ _ _ _ _ _ _ _ _ _ _ _ _ _ _ _ _ _ _ _ _ _ _ _ _ _]
          dyn-events: _ -> [_ _ _ _ _ _ _ _ _ _ _ _ _ _ _ _ _ _ _ _ _ _ _ _ _ _ _ _ _ _ _ _ _ _ _ _ _ _ _ _ _ _ _]
          timeout: 10 -> [_ _ _ _ _ _ _ _ _ _ _ _ _ _ _ _ _ _ _ _ _ _ _ _ _ _ _ _ _ _ _ _ _ _ _ _ _ _ _ _ _ _ _]
          tunnel: w4421 -> [_ w4477 w4522 w4547 w4639 w4678 w4798 w4833 w5013 w5046 w5152 w5179 w5282 w5317 w5412 w5447 w5542 w5577 w5672 w5707 w5804 w5841 w5934 w5967 w6063 w6092 w6289 w6327 w6422 w6457 w6552 w6587 w6715 w6734 w6769 w6866 w6901 w7085 w7116 w7146 w7310 w7381 w7552]
          tunnel: w4420 -> [_ w4476 w4521 w4546 w4640 w4677 w4797 w4832 w5012 w5047 w5151 w5178 w5281 w5316 w5411 w5446 w5541 w5576 w5671 w5706 w5803 w5842 w5933 w5968 w6062 w6091 w6288 w6326 w6421 w6456 w6551 w6586 w6714 w6733 w6768 w6865 _ w7084 w7115 w7145 w7309 w7380 w7551]
          tunnel: [errorcluster {"status"=FALSE, "code"=0, "source"=""} ("error out") w4458 w4512 w4552 w4637 w4676 errorcluster {"status"=FALSE, "code"=0, "source"=""} ("error out") w4831 w5010 w5044 w5150 w5173 w5280 w5313 w5410 w5443 w5539 w5573 w5670 w5703 w5801 w5840 w5932 w5966 w6060 w6090 w6287 w6323 w6419 w6453 w6550 w6583 w6680 w6731 w6765 w6864 w6905 w7075 w7123 w7173 w7301 w7379 w7550] -> w4418
          tunnel: ["" "ST101 扫码请求错误" "ST10 右扫码请求错误" "ST10 数据读取错误" "ST201 扫码请求错误" "ST201 数据读取错误" "ST202 扫码请求错误" "ST202 数据保存请求错误" "ST301 扫码请求错误" "ST301 数据读取错误" "ST302 扫码请求错误" "ST302 数据读取错误" "ST303 扫码请求错误" "ST303 数据读取错误" "ST401 扫码请求错误" "ST401 数据读取错误" "ST402 扫码请求错误" "ST402 数据读取错误" "ST501 扫码请求错误" "ST501 数据读取错误" "ST502 扫码请求错误" "ST502 数据读取错误" "ST503 扫码请求错误" "ST503 数据读取错误" "ST504 扫码请求错误" "ST504 数据读取错误" "ST601 扫码请求错误" "ST601 数据读取错误" "ST602 扫码请求错误" "ST602 数据读取错误" "ST603 扫码请求错误" "ST603 数据读取错误" "ST70 数据读取错误" "ST80 扫码请求错误" "ST80 数据读取错误" "ST901 扫码请求错误" "ST901 数据读取错误" "ST901 编码请求错误" "ST902 扫码请求错误" "ST902 数据读取错误" "ST100 数据读取错误" "查询数据库失败" "Rework失败"] -> w4417
          event Timeout {
            n583 = event-data() -> ()  [unwired: 1 in, 3 out]
          }
          event "ST101扫码请求（事件）": Value Change {
            w4437 = path "D:/op10" ("路径")
            # "判断数据库中有无该条码"
            n584 = event-data() -> ()  [unwired: 1 in, 1 out]
            n585 = List Folder(path=w4437) -> (filenames=w4436:string[])  [unwired: 3 in, 3 out]
            n586 = for {
              tunnel: w4436 -> [w4481] mode=indexing
              tunnel: w4437 -> [w4482]
              n587 = Build Path(base path=w4482, name or relative path=w4481) -> (appended path=w4479:path)
              n588 = Delete(path (use dialog)=w4479, entire hierarchy (F)=TRUE ("整个层次结构(F)")) -> ()  [unwired: 3 in, 3 out]
            }
            n589 = local read "101二维码"() -> (w4442:string)
            n590 = Concatenate Strings("Where QRCode='" ("查询语句"), w4442, "'" ("字符串")) -> (w4452:string)
            n591 = call "SQL_Select.vi"("表名"="Online", "error in (no error)"=w4476, "查询语句"=w4452, "查询条件"=TRUE, "connection reference"=w4477) -> ("error out"=w4453:errorcluster, "数据"=w4471:string[][], "connection reference out"=w4454:T5)  [unwired: 4 in]
            n592 = call "SQL_Select.vi"("表名"="Offline", "error in (no error)"=w4453, "查询语句"=w4452, "查询条件"=TRUE, "connection reference"=w4454) -> ("error out"=w4451:errorcluster, "数据"=w4447:string[][], "connection reference out"=w4450:T5)  [unwired: 4 in]
            n593 = Matrix Size(0:w4447) -> (1:w4448:i32)  [unwired: 1 out]
            n594 = Matrix Size(0:w4471) -> (1:w4470:i32)  [unwired: 1 out]
            n595 = local read "101打码等级"() -> (w4441:string)
            n596 = Equal?(x=w4448, y=0) -> (x = y?=w4445:bool)
            n597 = Equal?(x=w4470, y=0) -> (x = y?=w4446:bool)
            n598 = And(x=w4445, y=w4446) -> (x .and. y?=w4444:bool)
            n599 = case shown="真" w4444 {
              tunnel: w4450 -> [_ w4502]
              tunnel: w4451 -> [w4484 w4501]
              tunnel: w4442 -> [_ w4499]
              tunnel: ["2" ("左扫码请求回复") w4494] -> w4440
              tunnel: [w4484 w4488] -> w4458
              tunnel: w4441 -> [_ w4489]
              tunnel: [errorcluster {"status"=FALSE, "code"=0, "source"=""} ("error out") errorcluster {"status"=FALSE, "code"=0, "source"=""} ("error out")] -> w4439
              frame False {
              }
              frame True {
                # "该条码数据插入Online中"
                n600 = local read "产品型号10"() -> (w4486:string)
                n601 = Format Date/Time String(time format string (%c)="%Y-%m-%d_%H:%M" ("时间格式字符串(%c)")) -> (date/time string=w4492:string)  [unwired: 2 in]
                n602 = Insert Into Array(array=string[] [] ("数组"), index=0 ("索引"), new element #1=w4499, new element #2=w4492, new element #3="101" ("新元素/子数组"), new element #4="OK" ("新元素/子数组"), new element #5=w4489, new element #6=w4486) -> (w4496:string[])
                n603 = call "SQL_Insert.vi"("表名"="Online", "error in (no error)"=w4501, "值"=w4496, "列名"=string[] ["QRCode", "Online_Time", "Last_Station", "Last_Result", "Marking_Upclass", "ProductType"], "connection reference"=w4502) -> ("error out"=w4488:errorcluster)  [unwired: 5 in, 1 out]
                n604 = case shown="无错误" w4488 {
                  tunnel: ["1" ("左扫码请求回复") "3" ("左扫码请求回复")] -> w4494
                  frame No Error {
                  }
                  frame Error {
                  }
                }
              }
            }
            "扫码请求回复101" <- w4440
            n605 = property on="101扫码回复写入" class="Bool (严格)"(error in=w4439, "Value"=TRUE ("101扫码回复写入")) -> ()  [unwired: 1 in, 2 out]
            n606 = Get Date/Time String(want seconds? (F)=TRUE ("需要秒？(F)")) -> (time string=w4466:string)  [unwired: 2 in, 1 out]
            n607 = Format Date/Time String(time format string (%c)="%Y-%m-%d" ("时间格式字符串(%c)")) -> (date/time string=w4467:string)  [unwired: 2 in]
            n608 = Insert Into Array(array=string[] [] ("数组"), index=0 ("索引"), new element #1=w4467, new element #2=w4466, new element #3=w4441, new element #4=w4442) -> (w4463:string[])
            n609 = Insert Into Array(array=string[][] [] ("数组"), index (row)=0 ("索引 (行)"), new element=w4463) -> (w4460:string[][])  [unwired: 1 in]
            n610 = Transpose 2D Array(2D array=w4460) -> (transposed array=w4459:string[][])
            n611 = property on="ST101_DATA" class="MCListbox (严格)"("ItemNames"=w4459) -> ()  [unwired: 2 in, 2 out]
            "ST101扫码请求（事件）" <- FALSE ("ST10左扫码请求")
          }
          event "ST102扫码请求（事件）": Value Change {
            n612 = event-data() -> ()  [unwired: 1 in, 1 out]
            n613 = local read "102二维码"() -> (w4510:string)
            n614 = Concatenate Strings("Where QRCode='" ("查询语句"), w4510, "'" ("字符串")) -> (w4515:string)
            n615 = call "SQL_Select.vi"("要读取的列名"=string[] ["Last_Station", "Last_Result"], "表名"="Online", "error in (no error)"=w4521, "查询语句"=w4515, "查询条件"=TRUE, "connection reference"=w4522) -> ("error out"=w4512:errorcluster, "数据"=w4514:string[][])  [unwired: 3 in, 1 out]
            n616 = case shown="无错误" w4512 {
              tunnel: w4514 -> [w4530 _]
              tunnel: ["1" ("右扫码请求回复") "2" ("右扫码请求回复")] -> w4509
              tunnel: [w4525 w4532] -> w4508
              tunnel: [w4524 w4532] -> w4507
              tunnel: [errorcluster {"status"=FALSE, "code"=0, "source"=""} ("错误输出") errorcluster {"status"=FALSE, "code"=0, "source"=""} ("错误输出")] -> w4505
              frame No Error {
                n617 = Index Array(array=w4530, index (row)=0 ("索引 (行)")) -> (element=w4527:string[])  [unwired: 1 in]
                n618 = Index Array(array=w4527, index #1=0 ("索引 (行)")) -> (element #1=w4524:string, element #2=w4525:string)  [unwired: 1 in]
              }
              frame Error {
                w4532 = ""
              }
            }
            "扫码请求回复102" <- w4509
            "上一站号(10)" <- w4507
            "上一站结果(10)" <- w4508
            n619 = property on="102数据回复写入" class="Bool (严格)"(error in=w4505, "Value"=TRUE ("102数据回复写入")) -> ()  [unwired: 1 in, 2 out]
            "ST102扫码请求（事件）" <- FALSE ("ST10右扫码请求（事件）")
          }
          event "ST102数据读取（事件）": Value Change {
            w4543 = 0 ("索引 (行)")
            n620 = event-data() -> ()  [unwired: 1 in, 1 out]
            n621 = local read "101二维码"() -> (w4536:string)
            n622 = Concatenate Strings("Where QRCode='" ("查询语句"), w4536, "'" ("字符串")) -> (w4545:string)
            n623 = call "SQL_Select.vi"("要读取的列名"=string[] ["Rework_Status"], "表名"="Online", "error in (no error)"=w4546, "查询语句"=w4545, "查询条件"=TRUE, "connection reference"=w4547) -> ("error out"=w4538:errorcluster, "数据"=w4544:string[][], "connection reference out"=w4539:T5)  [unwired: 3 in]
